vi "markov chains.vi"(5 "p12":dbl, 9 "p21":dbl) -> (8 "bit":bool)   [LabVIEW 2017]
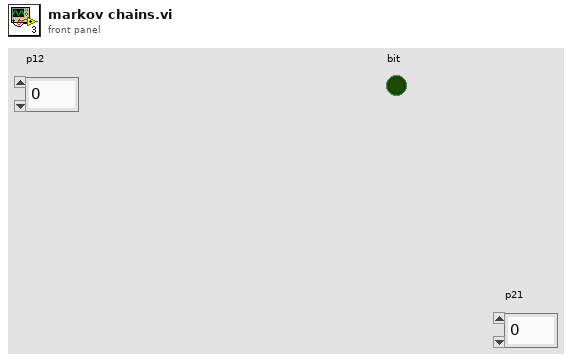
[diagram p1: front panel]
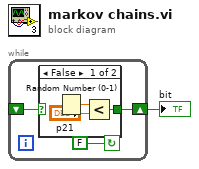
[diagram p0: block diagram]
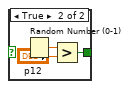
[diagram p2: hidden frame]
diagram:
  n1 = while {
    shift-right: [w3] -> w1
    shift-left: _ -> [w2]
    stop <- FALSE continue-if-true
    n2 = case shown="False" w2 {
      tunnel: [w5 w10] -> w3
      frame False {
        n3 = Random Number (0-1)() -> (number: 0 to 1=w7:dbl)
        n4 = Less?(x=w7, y="p21") -> (x < y?=w5:bool)
      }
      frame True {
        n5 = Random Number (0-1)() -> (number: 0 to 1=w9:dbl)
        n6 = Greater?(x=w9, y="p12") -> (0:w10:bool)
      }
    }
  }
  "bit" <- w1
